vi "Spartan Event Log.vi"(4 "Force Archive? (f)":bool, 5 "error in (no error)":errorcluster, 6 "username (\"\")":string, 7 "module (\"\")":string, 8 "message (\"\")":string) -> (0 "error out":errorcluster)   [LabVIEW 2011]
uses:
  errorlog types.ctl
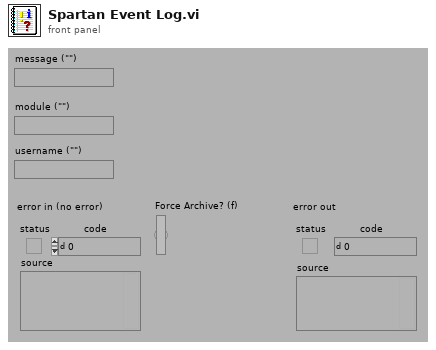
[diagram p1: front panel]
types:
  T1 = typedef "errorlog types.ctl" = enum16{"Information", "Warning", "Error"}
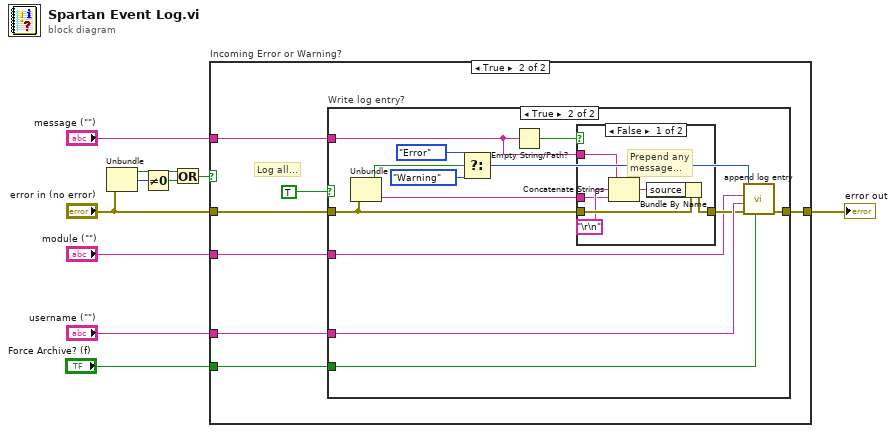
[diagram p0: block diagram]
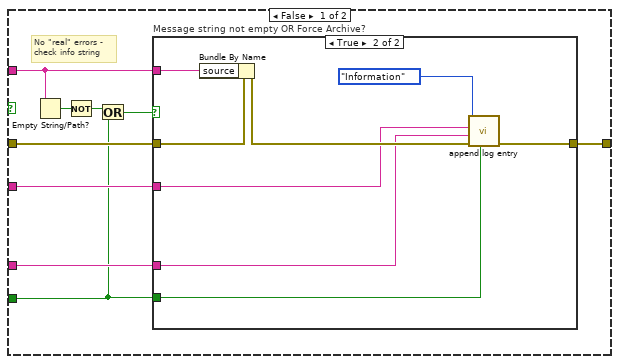
[diagram p2: hidden frame]
diagram:
  n1 = Unbundle("error in (no error)") -> ("status"=w5:bool, "code"=w4:i32)  [unwired: 1 out]
  n2 = Not Equal To 0?(x=w4) -> (x != 0?=w3:bool)
  n3 = Or(x=w5, y=w3) -> (x .or. y?=w2:bool)
  n4 = case "Incoming Error or Warning?" shown="True" w2 {
    tunnel: "message (\"\")" -> [w19 w34]
    tunnel: [w18 w35] -> w7
    tunnel: "error in (no error)" -> [w17 w31]
    tunnel: "module (\"\")" -> [w16 w33]
    tunnel: "username (\"\")" -> [w15 w32]
    tunnel: "Force Archive? (f)" -> [w12 w30]
    frame False {
      # "No \"real\" errors -\ncheck info string"
      n5 = Empty String/Path?(string/path=w19) -> (empty?=w14:bool)
      n6 = Not(x=w14) -> (.not. x?=w11:bool)
      n7 = Or(x=w11, y=w12) -> (x .or. y?=w13:bool)
      n8 = case "Message string not empty OR Force Archive?" shown="True" w13 {
        tunnel: w17 -> [w20 w27]
        tunnel: w19 -> [_ w26]
        tunnel: [w20 w28] -> w18
        tunnel: w16 -> [_ w21]
        tunnel: w15 -> [_ w24]
        tunnel: w12 -> [_ w23]
        frame False {
          # "Nothing to write ... move on"
        }
        frame True {
          n9 = Bundle By Name(cluster=w27, "source"=w26) -> (w25:errorcluster)
          n10 = call "append log entry.vi"("Force Archive? (f)"=w23, "error in (no error)"=w25, "Username (\"\")"=w24, "Module Name (\"\")"=w21, "Error Type (Information)"=errorlog_types."Information" ("Error Types")) -> ("error out"=w28:errorcluster)  [unwired: 5 out]
        }
      }
    }
    frame True {
      # "Log all..."
      n11 = case "Write log entry?" shown="True" TRUE {
        tunnel: [w36 w46] -> w35
        tunnel: w31 -> [w36 w41]
        tunnel: w33 -> [_ w37]
        tunnel: w30 -> [_ w45]
        tunnel: w34 -> [_ w39]
        tunnel: w32 -> [_ w43]
        frame False {
          # "Nothing to write ... move on"
        }
        frame True {
          n12 = Unbundle(w41) -> ("status"=w49:bool, "source"=w42:string)  [unwired: 1 out]
          n13 = Select(t=errorlog_types."Error" ("Error Types"), s=w49, f=errorlog_types."Warning" ("Error Types")) -> (s? t:f=w44:T1)
          n14 = Empty String/Path?(string/path=w39) -> (empty?=w38:bool)
          n15 = case shown="False" w38 {
            tunnel: w42 -> [w50 _]
            tunnel: w41 -> [w55 w56]
            tunnel: [w54 w56] -> w40
            tunnel: w39 -> [w51 _]
            frame False {
              # "Prepend any\nmessage..."
              n16 = Concatenate Strings(w51, "\r\n", w50) -> (w53:string)
              n17 = Bundle By Name(cluster=w55, "source"=w53) -> (w54:errorcluster)
            }
            frame True {
            }
          }
          n18 = call "append log entry.vi"("Force Archive? (f)"=w45, "error in (no error)"=w40, "Username (\"\")"=w43, "Module Name (\"\")"=w37, "Error Type (Information)"=w44) -> ("error out"=w46:errorcluster)  [unwired: 5 out]
        }
      }
    }
  }
  "error out" <- w7
